vi "Create Indices (U32).vi"(8 "error in":errorcluster[](array[cluster]), 11 "connection in":refnum<k13>[](array[refnum])) -> (0 "error out":errorcluster[](array[cluster]), 1 "Indices":i32[](array[numeric]), 2 "Output Words":u32[](array[numeric]), 3 "connection out":refnum<k13>[](array[refnum]))   [LabVIEW 2011]
uses:
  GlobalVariables.vi
panel:
  out "Count":i32
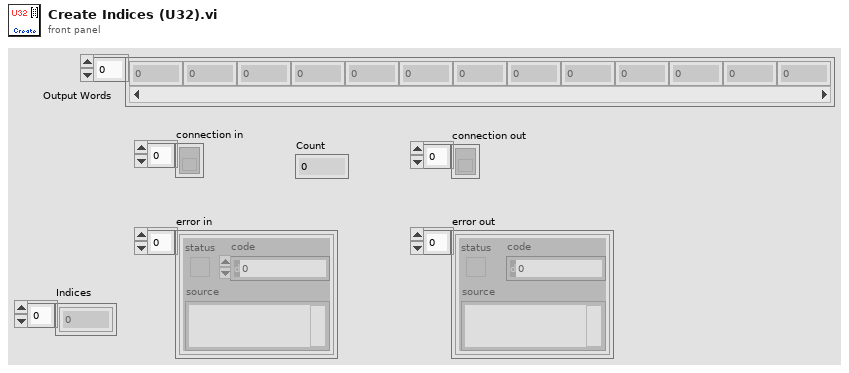
[diagram p1: front panel]
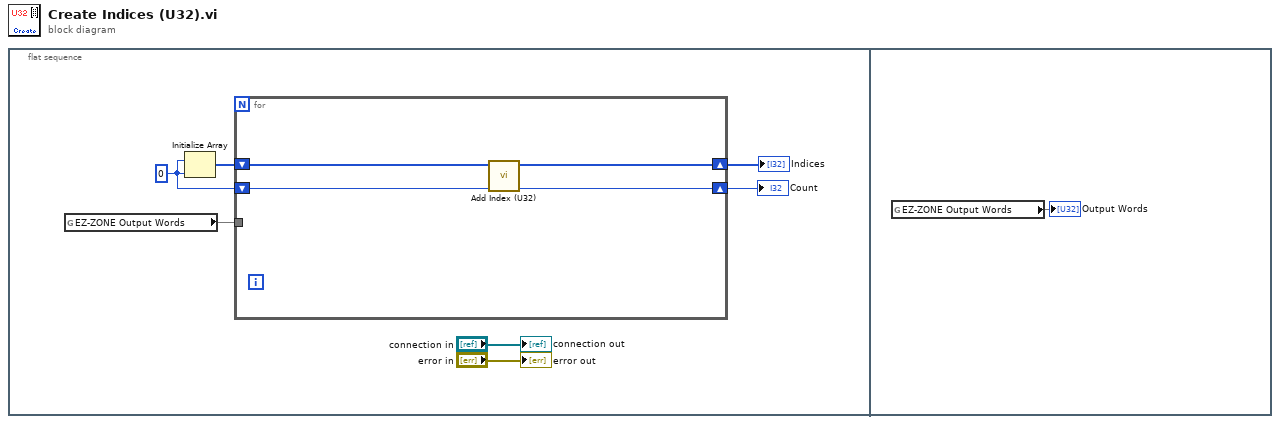
[diagram p0: block diagram]
diagram:
  n1 = flat-sequence {
    frame #0 {
      w2 = 0 ("dimension size")
      n2 = global read "GlobalVariables.vi" "EZ-ZONE Output Words"() -> (w1)
      n3 = Initialize Array(w2, w2) -> (w4:i32[])
      n4 = for {
        shift-right: [w11] -> w5
        shift-left: w4 -> [w8]
        shift-right: [w10] -> w3
        shift-left: w2 -> [w9]
        tunnel: w1 -> [_]
        n5 = call "Add Index (U32).vi"("Count"=w9, "Indices Input"=w8) -> ("Count+1"=w10:i32, "Indices Output"=w11:i32[])  [unwired: 7 in]
      }
      "Indices" <- w5
      "Count" <- w3
      "connection out" <- "connection in"
      "error out" <- "error in"
    }
    frame #1 {
      n6 = global read "GlobalVariables.vi" "EZ-ZONE Output Words"() -> (→"Output Words")
    }
  }
